vi "flash_vna_temperature.vi"(2 "error in":errorcluster) -> (0 "error out":errorcluster, 1 "File":path)   [LabVIEW 2013]
doc: "Runs before the main program, to ensure that VNA is switched on and the temperature log file is loaded"
panel:
  in  "Boolean 3":bool=TRUE
  in  "Path":path=path "Z:/18-09-21/CH5 T 18-09-21.log"
  in  "Boolean 2":bool
  in  "Boolean":bool
  # "Load CH5 T from most recent log file"
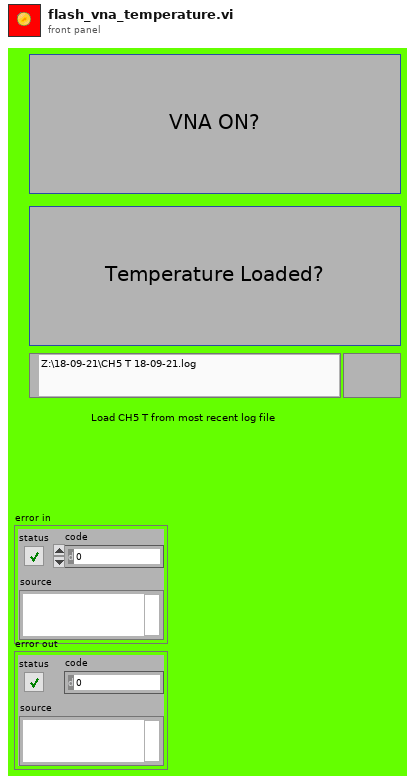
[diagram p1: front panel]
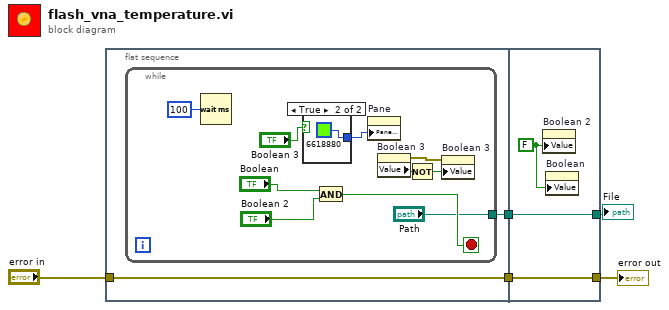
[diagram p0: block diagram]
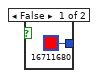
[diagram p2: hidden frame]
diagram:
  n1 = flat-sequence {
    tunnel: [w7] -> w4
    tunnel: "error in" -> [w6]
    tunnel: [w6] -> w2
    tunnel: [w22] -> w5
    tunnel: w4 -> [w22]
    tunnel: [w20] -> w1
    tunnel: w2 -> [w20]
    frame #0 {
      n2 = while {
        tunnel: ["Path"] -> w7
        stop <- w15 stop-if-true
        n3 = Wait (ms)(milliseconds to wait=u32 100) -> ()  [unwired: 1 out]
        n4 = case shown="True" "Boolean 3" {
          tunnel: [u32 16711680 u32 6618880] -> w14
          frame False {
          }
          frame True {
          }
        }
        n5 = And(x="Boolean", y="Boolean 2") -> (x .and. y?=w15:bool)
        n6 = property on="Pane" class="Pane"("PaneColor"=w14) -> ()  [unwired: 2 in, 2 out]
        n7 = property on="Boolean 3" class="Bool (strict)"() -> (error out=w13:errorcluster, "Value"=w12:bool)  [unwired: 2 in, 1 out]
        n8 = Not(x=w12) -> (.not. x?=w11:bool)
        n9 = property on="Boolean 3" class="Bool (strict)"(error in=w13, "Value"=w11) -> ()  [unwired: 1 in, 2 out]
      }
    }
    frame #1 {
      w21 = FALSE ("Boolean 2")
      n10 = property on="Boolean 2" class="Bool (strict)"("Value"=w21) -> ()  [unwired: 2 in, 2 out]
      n11 = property on="Boolean" class="Bool (strict)"("Value"=w21) -> ()  [unwired: 2 in, 2 out]
    }
  }
  "File" <- w5
  "error out" <- w1
